vi "Msg Send Message.vi"   [LabVIEW 2014]
doc: "Send a message to the specified message queue (or event structure). This function awaits a response from the recipient which should be sent with Msg Send Response.vi.\n\nThis is part of the Msg suite, intended to make messaging architectures in LabVIEW\nSee the template \"Message Based Application Template.vi\" for normal usage.\n\nCopyright 2005-2016 Jason Sommerville\n\nSends a response to the original sender of a message (sent via Msg Send Message). It should form bookends with Msg Get Message in the message handling loop.\n\nThis is part of the Msg suite, intended to make messaging architectures in LabVIEW\nSee the template \"Message Based Application Template.vi\" for normal usage.\n\nCopyright 2005-2016 Jason Sommerville\n\nThis VI may be freely used, modified or distributed under the BSD license."
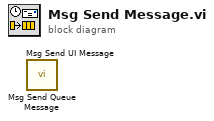
[diagram p0: block diagram]
diagram:
  n1 = call "Msg Send Queue Message.vi"() -> ()  [unwired: 6 in, 4 out]
  n2 = call "Msg Send UI Message.vi"() -> ()  [unwired: 6 in, 4 out]
